vi "Main.vi"() -> ()   [LabVIEW 2022 SP3]
doc: "该连续测量范例项目在队列消息处理器模板的基础上实现。\n\n事件处理循环负责按用户界面操作生成对应的消息。\n\n消息处理循环负责对事件处理循环或其他消息生成的消息进行处理。 其中还包括用于采集和记录消息处理循环的子VI，以及用于更新图表的循环。"
uses:
  Settings/Settings.ctl
  Acquisition/Hardware Configuration.ctl
  Acquisition/Signal Type.ctl
  Logging/Logging Configuration.ctl
  controls/UI Data.ctl
  controls/UI State.ctl
  support/Message Queue/Enqueue Message (Single).vi
  support/Message Queue/Enqueue Message (Array).vi
  <vilib>/Utility/error.llb/Error Cluster From Error Code.vi
  <vilib>/ErrorRing/Error Ring.xnode
  Acquisition/Acquisition.lvlib
  Logging/Logging.lvlib
  Settings/Settings.lvlib
  support/User Event - Stop/User Event - Stop.lvlib
  support/Message Queue/Message Queue.lvlib
  Settings/Settings Dialog.vi
panel:
  out "数据":waveform(dbl)[](graph)
  in  "设置":bool
  in  "开始":bool
  in  "停止":bool
  out "状态":string
  in  "退出":bool
  # "连续测量数据记录器"
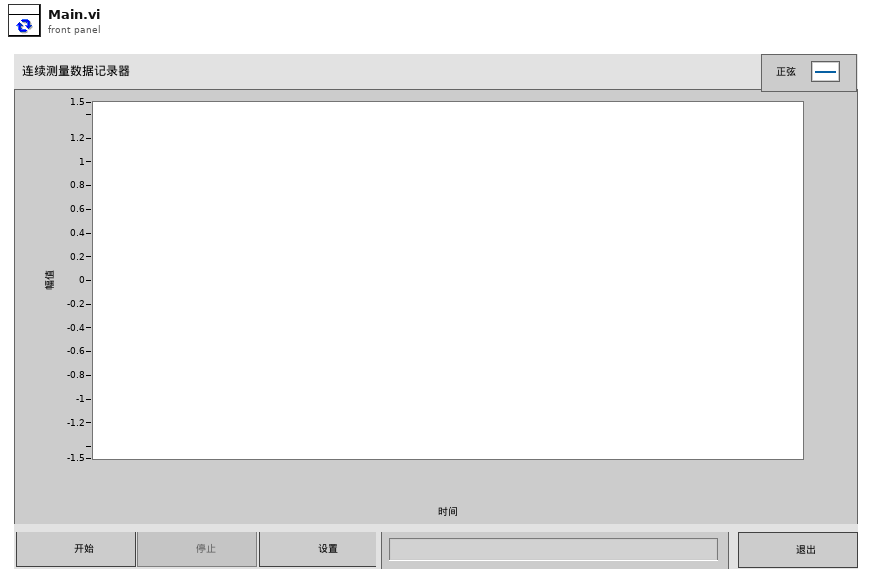
[diagram p1: front panel]
types:
  T1 = typedef "UI State.ctl" = enum16{"Idle", "Acquiring and Logging", "Waiting for Exit", "Waiting for Exit (Acq Stopped)", "Waiting for Exit (Log Stopped)", "Waiting for Stop", "Waiting for Stop (Acq Stopped)", "Waiting for Stop (Log Stopped)"}
  T2 = typedef "UI Data.ctl" = cluster{"开始引用":refnum<vi>, "停止引用":refnum<vi>, "设置引用":refnum<vi>, "退出引用":refnum<vi>, "状态引用":refnum<vi>, "数据引用":refnum<vi>}
  T3 = typedef "Settings.lvlib/Settings.ctl" = cluster{"硬件配置":T4, "记录配置":T6}
  T4 = typedef "Acquisition.lvlib/Hardware Configuration.ctl" = cluster{"硬件引用句柄<替换此项>":string, "信号类型<替换该项>":T5}
  T5 = typedef "Acquisition.lvlib/Signal Type.ctl" = enum16{"Sine Wave", "Square with Noise"}
  T6 = typedef "Logging.lvlib/Logging Configuration.ctl" = cluster{"记录文件基路径":path, "TDMS文件引用":refnum<k34>}
  T7 = typedef "Message Queue.lvlib/All Message Queues.ctl" = cluster{"UI":refnum<queue>, "采集":refnum<queue>, "记录":refnum<queue>}
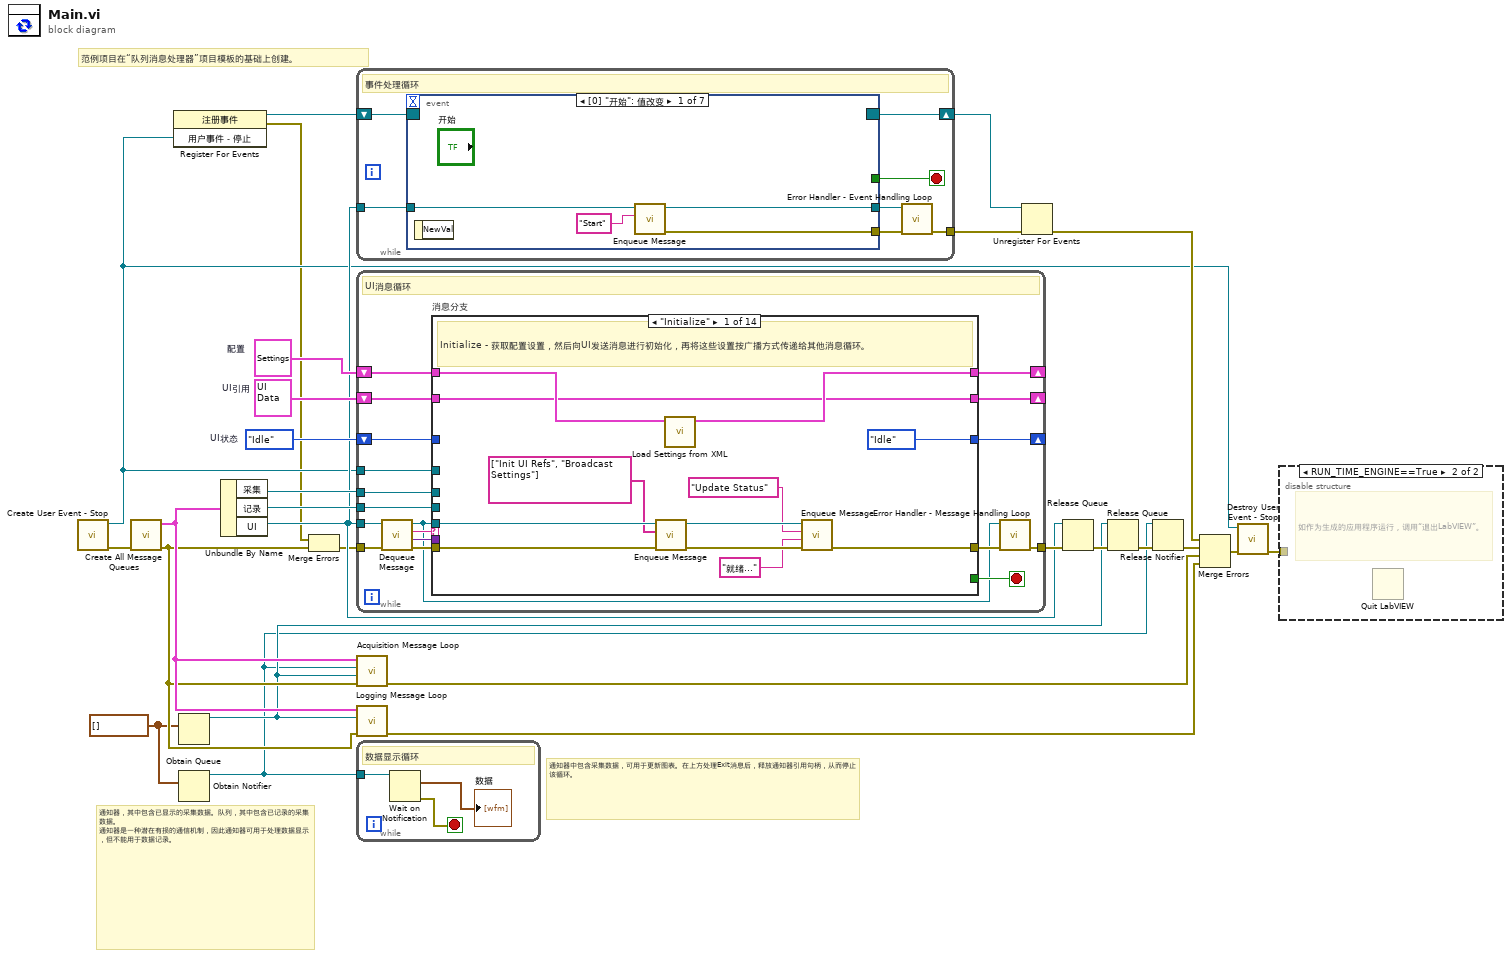
[diagram p0: block diagram]
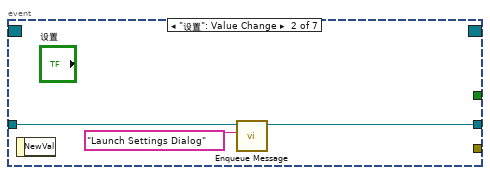
[diagram p3: hidden frame]
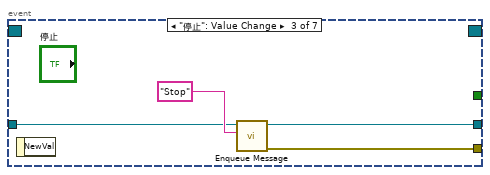
[diagram p4: hidden frame]
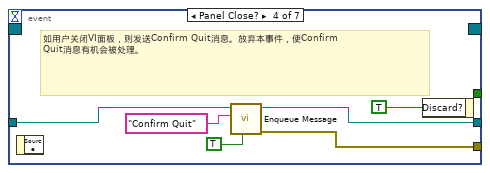
[diagram p5: hidden frame]
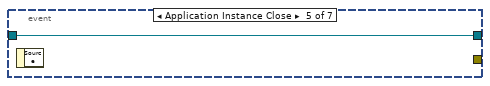
[diagram p6: hidden frame]
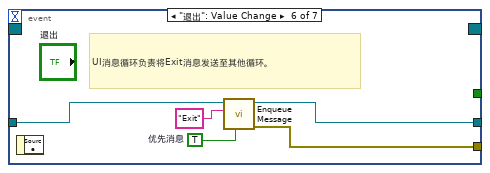
[diagram p7: hidden frame]
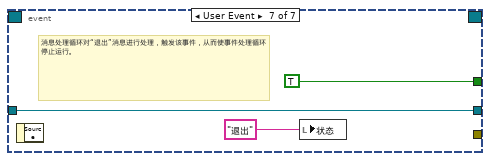
[diagram p8: hidden frame]
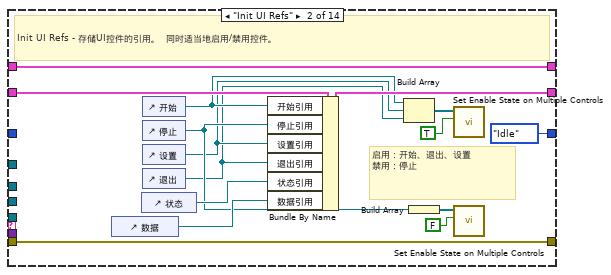
[diagram p9: hidden frame]
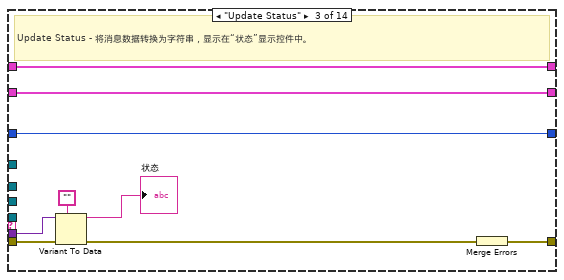
[diagram p10: hidden frame]
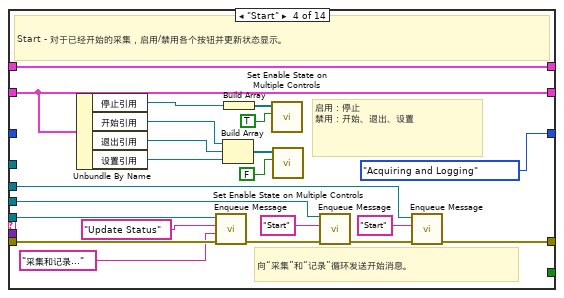
[diagram p11: hidden frame]
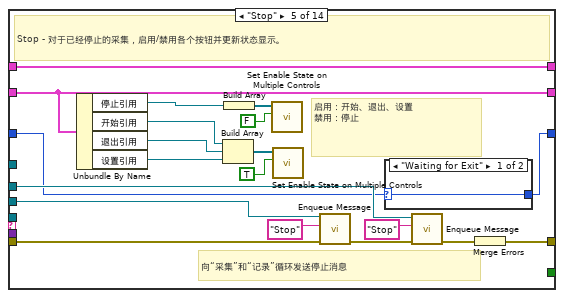
[diagram p12: hidden frame]
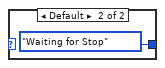
[diagram p13: hidden frame]
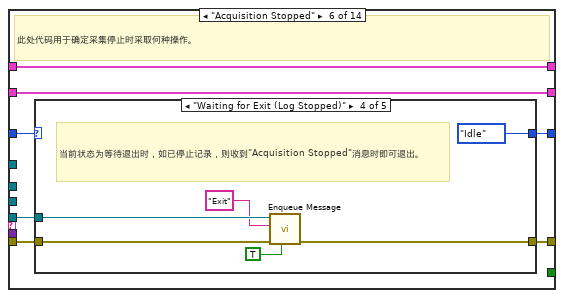
[diagram p14: hidden frame]
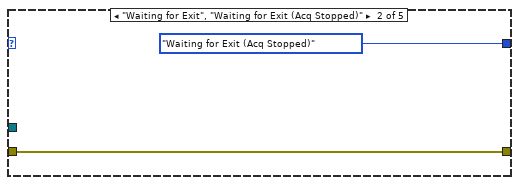
[diagram p16: hidden frame]
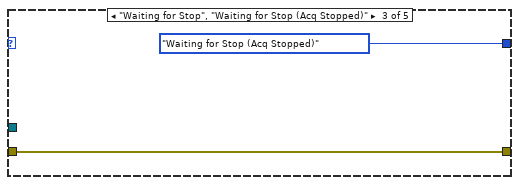
[diagram p17: hidden frame]
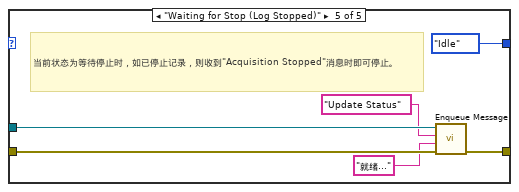
[diagram p18: hidden frame]
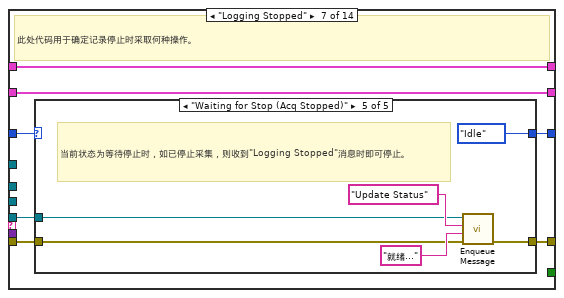
[diagram p19: hidden frame]
diagram:
  w14 = UI_State."Idle"  # UI状态
  w5 = waveform(dbl)[] []
  w17 = T2 {"开始引用"=refnum, "停止引用"=refnum, "设置引用"=refnum, "退出引用"=refnum, "状态引用"=refnum, "数据引用"=refnum}  # UI引用
  w20 = T3 {"硬件配置"={"硬件引用句柄<替换此项>"="", "信号类型<替换该项>"=enum."Sine Wave"}, "记录配置"={"记录文件基路径"=path "", "TDMS文件引用"=refnum}}  # 配置
  # "范例项目在“队列消息处理器”项目模板的基础上创建。"
  # "通知器，其中包含已显示的采集数据。队列，其中包含已记录的采集数据。  通知器是一种潜在有损的通信机制，因此通知器可用于处理数据显示，但不能用于数据记录。"
  # "通知器中包含采集数据，可用于更新图表。在上方处理Exit消息后，释放通知器引用句柄，从而停止该循环。"
  n1 = call "Create User Event - Stop.vi"() -> ("error out"=w24:cluster{"状态":bool, "代码":i32, "源":string}, "用户事件－停止"=w3:refnum<user-event>)  [unwired: 10 in]
  n2 = call "Create All Message Queues.vi"("error in (no error)"=w24) -> ("error out"=w21:cluster{"状态":bool, "代码":i32, "源":string}, "消息队列输出"=w23:T7)  [unwired: 9 in]
  n3 = register-events(w3) -> (reference out=w4:refnum<event-registration>, error out=w1:errorcluster)  [unwired: 2 in]
  n4 = Obtain Queue(element data type=w5) -> (queue out=w7:refnum<queue>)  [unwired: 4 in, 2 out]
  n5 = Obtain Notifier(notification data type=w5) -> (notifier out=w6:refnum<notifier>)  [unwired: 3 in, 2 out]
  n6 = Unbundle By Name(w23) -> ("采集"=w16:refnum<queue>, "记录"=w15:refnum<queue>, "UI"=w12:refnum<queue>)
  n7 = Merge Errors(w1, w21) -> (w2:errorcluster)
  n8 = while {
    tunnel: w12 -> [w33]
    tunnel: [w30] -> w26
    shift-right: [w32] -> w18
    shift-left: w4 -> [w34]
    stop <- w31 stop-if-true
    # "事件处理循环"
    n9 = event shown="[0] \"开始\": 值改变" {
      selector: w34 -> [_ _ _ _ _ _ _]
      dyn-events: [_ _ _ _ _ _ _] -> w32
      timeout: _ -> [_ _ _ _ _ _ _]
      tunnel: [_ _ _ _ _ _ TRUE ("Discard?")] -> w31
      tunnel: w33 -> [w38 w40 w44 w49 w52 w54 w58]
      tunnel: [w36 _ w43 w47 _ w57 _] -> w29
      tunnel: [w35 w39 w42 w48 w52 w53 w58] -> w28
      event "开始": Value Change {
        n10 = event-data() -> ()  [unwired: 1 in, 1 out]
        n11 = call-poly "Enqueue Message.vi"("消息"="Start" ("Message"), "消息队列"=w38) -> ("error out"=w36:cluster{"状态":bool, "代码":i32, "源":string}, "消息队列副本"=w35:refnum<queue>)  [unwired: 8 in]
      }
      event "设置": Value Change {
        n12 = event-data() -> ()  [unwired: 1 in, 1 out]
        n13 = call-poly "Enqueue Message.vi"("消息"="Launch Settings Dialog" ("Message"), "消息队列"=w40) -> ("消息队列副本"=w39:refnum<queue>)  [unwired: 8 in, 1 out]
      }
      event "停止": Value Change {
        n14 = event-data() -> ()  [unwired: 1 in, 1 out]
        n15 = call-poly "Enqueue Message.vi"("消息"="Stop" ("Message"), "消息队列"=w44) -> ("error out"=w43:cluster{"状态":bool, "代码":i32, "源":string}, "消息队列副本"=w42:refnum<queue>)  [unwired: 8 in]
      }
      event Panel Close? {
        # "如用户关闭VI面板，则发送Confirm Quit消息。放弃本事件，使Confirm Quit消息有机会被处理。"
        n16 = event-data() -> ()  [unwired: 1 in, 1 out]
        n17 = call-poly "Enqueue Message.vi"("优先消息？ (F)"=TRUE ("Priority Message? (F)"), "消息"="Confirm Quit" ("Message"), "消息队列"=w49) -> ("error out"=w47:cluster{"状态":bool, "代码":i32, "源":string}, "消息队列副本"=w48:refnum<queue>)  [unwired: 7 in]
        n18 = event-data ("Event Filter Node")("Discard?"=TRUE) -> ()  [unwired: 1 in, 1 out]
      }
      event Application Instance Close {
        n19 = event-data() -> ()  [unwired: 1 in, 1 out]
      }
      event "退出": Value Change {
        w55 = TRUE  # 优先消息
        # "UI消息循环负责将Exit消息发送至其他循环。"
        n20 = event-data() -> ()  [unwired: 1 in, 1 out]
        n21 = call-poly "Enqueue Message.vi"("优先消息？ (F)"=w55, "消息"="Exit" ("Message"), "消息队列"=w54) -> ("error out"=w57:cluster{"状态":bool, "代码":i32, "源":string}, "消息队列副本"=w53:refnum<queue>)  [unwired: 7 in]
      }
      event User Event {
        # "消息处理循环对“退出”消息进行处理，触发该事件，从而使事件处理循环停止运行。"
        n22 = event-data() -> ()  [unwired: 1 in, 1 out]
        n23 = local write "状态"("退出" ("Exit String")) -> ()
      }
    }
    n24 = call "Error Handler - Event Handling Loop.vi"("error in (no error)"=w29, "消息队列"=w28) -> ("错误输入副本"=w30:cluster{"状态":bool, "代码":i32, "源":string})  [unwired: 8 in, 1 out]
  }
  n25 = while {
    tunnel: w12 -> [w72]
    tunnel: w3 -> [w77]
    shift-right: [w71] -> _
    shift-left: w20 -> [w70]
    shift-right: [w68] -> _
    shift-left: w17 -> [w69]
    tunnel: w16 -> [w67]
    tunnel: w15 -> [w66]
    shift-right: [w61] -> _
    shift-left: w14 -> [w62]
    tunnel: w2 -> [w76]
    tunnel: [w65] -> w27
    stop <- w78 stop-if-true
    # "UI消息循环"
    n26 = call "Dequeue Message.vi"("error in (no error)"=w76, "消息队列"=w72) -> ("error out"=w75:cluster{"状态":bool, "代码":i32, "源":string}, "消息数据"=w73:variant, "消息"=w74:string, "消息队列副本"=w63:refnum<queue>)  [unwired: 6 in]
    n27 = case "消息分支" shown="\"Initialize\"" w74 {
      selector: w74 -> [_ _ _ _ _ _ _ _ _ _ _ _ _ w294]
      tunnel: w63 -> [w82 _ _ w136 _ w161 w186 _ w226 _ w247 _ _ _]
      tunnel: w75 -> [w81 w105 w113 w135 w155 w162 w187 w214 w228 w235 w246 w275 w292 _]
      tunnel: [w86 w105 w114 w118 w156 w159 w184 w220 w221 w238 w245 w285 w291 w293] -> w64
      tunnel: [_ _ _ _ _ _ _ _ _ _ _ TRUE _ _] -> w78
      tunnel: w73 -> [_ _ w112 _ _ _ _ _ _ w239 _ w273 _ _]
      tunnel: w77 -> [_ _ _ _ _ _ _ _ _ _ _ w286 _ _]
      tunnel: [w89 w104 w108 w134 w154 w165 w190 w218 w225 w243 w250 w284 w290 w297] -> w71
      tunnel: w70 -> [w90 w104 w108 w134 w154 w165 w190 w218 w229 w243 w250 w284 w290 w297]
      tunnel: w69 -> [w83 w103 w107 w131 w153 w164 w189 w212 w223 w242 w249 w283 w289 w296]
      tunnel: [w83 w100 w107 w131 w153 w164 w189 w212 w223 w242 w249 w283 w289 w296] -> w68
      tunnel: w67 -> [_ _ _ w117 w140 _ _ w211 _ _ _ w282 _ _]
      tunnel: w66 -> [_ _ _ w120 w143 _ _ w210 _ _ _ w281 _ _]
      tunnel: w62 -> [_ _ w106 _ w137 w163 w188 w209 w222 w237 w248 _ w288 w295]
      tunnel: [UI_State."Idle" ("UI State") UI_State."Idle" ("UI State") w106 UI_State."Acquiring and Logging" ("UI State") w138 w160 w185 w209 w222 w237 w244 UI_State."Idle" ("UI State") w288 w295] -> w61
      frame "Initialize" {
        # "Initialize - 获取配置设置，然后向UI发送消息进行初始化，再将这些设置按广播方式传递给其他消息循环。"
        n28 = call-poly "Enqueue Message.vi"("error in (no error)"=w81, "消息数组"=string[] ["Init UI Refs", "Broadcast Settings"], "消息队列"=w82) -> ("error out"=w88:cluster{"状态":bool, "代码":i32, "源":string}, "消息队列副本"=w87:refnum<queue>)  [unwired: 7 in]
        n29 = call "Load Settings from XML.vi"("设置输入"=w90) -> ("设置输出"=w89:T3)  [unwired: 9 in, 1 out]
        n30 = call-poly "Enqueue Message.vi"("error in (no error)"=w88, "消息数据"="就绪..." ("Ready..."), "消息"="Update Status" ("Message"), "消息队列"=w87) -> ("error out"=w86:cluster{"状态":bool, "代码":i32, "源":string})  [unwired: 6 in, 1 out]
      }
      frame "Init UI Refs" {
        # "启用：开始、退出、设置\n禁用：停止"
        # "Init UI Refs - 存储UI控件的引用。  同时适当地启用/禁用控件。"
        n31 = control-ref of="数据"() -> (w101:refnum<vi>)
        n32 = control-ref of="状态"() -> (w102:refnum<vi>)
        n33 = control-ref of="开始"() -> (w94:refnum<vi>)
        n34 = control-ref of="停止"() -> (w95:refnum<vi>)
        n35 = control-ref of="设置"() -> (w93:refnum<vi>)
        n36 = control-ref of="退出"() -> (w92:refnum<vi>)
        n37 = Bundle By Name(cluster=w103, "开始引用"=w94, "停止引用"=w95, "设置引用"=w93, "退出引用"=w92, "状态引用"=w102, "数据引用"=w101) -> (w100:T2)
        n38 = Build Array(w94, w93, w92) -> (w98:refnum<vi>[])
        n39 = Build Array(w95) -> (w97:refnum<vi>[])
        n40 = call "Set Enable State on Multiple Controls.vi"("启用？"=TRUE ("Enable?"), "控件"=w98) -> ()  [unwired: 10 in]
        n41 = call "Set Enable State on Multiple Controls.vi"("启用？"=FALSE ("Enable?"), "控件"=w97) -> ()  [unwired: 10 in]
      }
      frame "Update Status" {
        # "Update Status - 将消息数据转换为字符串，显示在“状态”显示控件中。"
        n42 = Variant To Data(error in=w113, type="" ("Empty String Constant"), Variant=w112) -> (data=→"状态":string, error out=w110:errorcluster)
        n43 = Merge Errors(w110) -> (w114:errorcluster)
      }
      frame "Start" {
        # "向“采集”和“记录”循环发送开始消息。"
        # "启用：停止\n禁用：开始、退出、设置"
        # "Start - 对于已经开始的采集，启用/禁用各个按钮并更新状态显示。"
        n44 = Unbundle By Name(w131) -> ("停止引用"=w126:refnum<vi>, "开始引用"=w125:refnum<vi>, "退出引用"=w124:refnum<vi>, "设置引用"=w123:refnum<vi>)
        n45 = call-poly "Enqueue Message.vi"("error in (no error)"=w135, "消息数据"="采集和记录..." ("Acquiring and Logging..."), "消息"="Update Status" ("Message"), "消息队列"=w136) -> ("error out"=w122:cluster{"状态":bool, "代码":i32, "源":string})  [unwired: 6 in, 1 out]
        n46 = Build Array(w125, w124, w123) -> (w129:refnum<vi>[])
        n47 = Build Array(w126) -> (w128:refnum<vi>[])
        n48 = call "Set Enable State on Multiple Controls.vi"("启用？"=TRUE ("Enable?"), "控件"=w128) -> ()  [unwired: 10 in]
        n49 = call "Set Enable State on Multiple Controls.vi"("启用？"=FALSE ("Enable?"), "控件"=w129) -> ()  [unwired: 10 in]
        n50 = call-poly "Enqueue Message.vi"("error in (no error)"=w122, "消息"="Start" ("Message"), "消息队列"=w120) -> ("error out"=w119:cluster{"状态":bool, "代码":i32, "源":string})  [unwired: 7 in, 1 out]
        n51 = call-poly "Enqueue Message.vi"("error in (no error)"=w119, "消息"="Start" ("Message"), "消息队列"=w117) -> ("error out"=w118:cluster{"状态":bool, "代码":i32, "源":string})  [unwired: 7 in, 1 out]
      }
      frame "Stop" {
        # "向“采集”和“记录”循环发送停止消息"
        # "启用：开始、退出、设置\n禁用：停止"
        # "Stop - 对于已经停止的采集，启用/禁用各个按钮并更新状态显示。"
        n52 = Unbundle By Name(w153) -> ("停止引用"=w148:refnum<vi>, "开始引用"=w147:refnum<vi>, "退出引用"=w146:refnum<vi>, "设置引用"=w145:refnum<vi>)
        n53 = Build Array(w147, w146, w145) -> (w151:refnum<vi>[])
        n54 = Build Array(w148) -> (w150:refnum<vi>[])
        n55 = call "Set Enable State on Multiple Controls.vi"("启用？"=FALSE ("Enable?"), "控件"=w150) -> ()  [unwired: 10 in]
        n56 = call "Set Enable State on Multiple Controls.vi"("启用？"=TRUE ("Enable?"), "控件"=w151) -> ()  [unwired: 10 in]
        n57 = call-poly "Enqueue Message.vi"("error in (no error)"=w155, "消息"="Stop" ("Message"), "消息队列"=w143) -> ("error out"=w142:cluster{"状态":bool, "代码":i32, "源":string})  [unwired: 7 in, 1 out]
        n58 = case shown="\"Waiting for Exit\"" w137 {
          selector: w137 -> [w157 _]
          tunnel: [w157 UI_State."Waiting for Stop" ("UI State")] -> w138
          frame "Waiting for Exit" {
          }
          frame Default {
          }
        }
        n59 = call-poly "Enqueue Message.vi"("error in (no error)"=w142, "消息"="Stop" ("Message"), "消息队列"=w140) -> ("error out"=w141:cluster{"状态":bool, "代码":i32, "源":string})  [unwired: 7 in, 1 out]
        n60 = Merge Errors(w141) -> (w156:errorcluster)
      }
      frame "Acquisition Stopped" {
        # "此处代码用于确定采集停止时采取何种操作。"
        n61 = case shown="\"Waiting for Exit (Log Stopped)\"" w163 {
          selector: w163 -> [w167 _ _ _ _]
          tunnel: w162 -> [w166 w169 w171 w177 w183]
          tunnel: w161 -> [_ _ _ w175 w180]
          tunnel: [w167 UI_State."Waiting for Exit (Acq Stopped)" ("UI State") UI_State."Waiting for Stop (Acq Stopped)" ("UI State") UI_State."Idle" ("UI State") UI_State."Idle" ("UI State")] -> w160
          tunnel: [w166 w169 w171 w176 w181] -> w159
          frame Default {
          }
          frame "Waiting for Exit", "Waiting for Exit (Acq Stopped)" {
          }
          frame "Waiting for Stop", "Waiting for Stop (Acq Stopped)" {
          }
          frame "Waiting for Exit (Log Stopped)" {
            # "当前状态为等待退出时，如已停止记录，则收到\"Acquisition Stopped\"消息时即可退出。"
            n62 = call-poly "Enqueue Message.vi"("优先消息？ (F)"=TRUE ("Priority Message? (F)"), "error in (no error)"=w177, "消息"="Exit", "消息队列"=w175) -> ("error out"=w176:cluster{"状态":bool, "代码":i32, "源":string})  [unwired: 6 in, 1 out]
          }
          frame "Waiting for Stop (Log Stopped)" {
            # "当前状态为等待停止时，如已停止记录，则收到\"Acquisition Stopped\"消息时即可停止。"
            n63 = call-poly "Enqueue Message.vi"("error in (no error)"=w183, "消息数据"="就绪..." ("Ready..."), "消息"="Update Status" ("Message"), "消息队列"=w180) -> ("error out"=w181:cluster{"状态":bool, "代码":i32, "源":string})  [unwired: 6 in, 1 out]
          }
        }
      }
      frame "Logging Stopped" {
        # "此处代码用于确定记录停止时采取何种操作。"
        n64 = case shown="\"Waiting for Stop (Acq Stopped)\"" w188 {
          selector: w188 -> [w192 _ _ _ _]
          tunnel: w187 -> [w191 w194 w196 w202 w205]
          tunnel: w186 -> [_ _ _ w200 w204]
          tunnel: [w192 UI_State."Waiting for Exit (Log Stopped)" ("UI State") UI_State."Waiting for Stop (Log Stopped)" ("UI State") UI_State."Idle" ("UI State") UI_State."Idle" ("UI State")] -> w185
          tunnel: [w191 w194 w196 w201 w203] -> w184
          frame Default {
          }
          frame "Waiting for Exit", "Waiting for Exit (Log Stopped)" {
          }
          frame "Waiting for Stop", "Waiting for Stop (Log Stopped)" {
          }
          frame "Waiting for Exit (Acq Stopped)" {
            # "当前状态为等待退出时，如已停止采集，则收到\"Logging Stopped\"消息时即可退出。"
            n65 = call-poly "Enqueue Message.vi"("优先消息？ (F)"=TRUE ("Priority Message? (F)"), "error in (no error)"=w202, "消息"="Exit", "消息队列"=w200) -> ("error out"=w201:cluster{"状态":bool, "代码":i32, "源":string})  [unwired: 6 in, 1 out]
          }
          frame "Waiting for Stop (Acq Stopped)" {
            # "当前状态为等待停止时，如已停止采集，则收到\"Logging Stopped\"消息时即可停止。"
            n66 = call-poly "Enqueue Message.vi"("error in (no error)"=w205, "消息数据"="就绪..." ("Ready..."), "消息"="Update Status" ("Message"), "消息队列"=w204) -> ("error out"=w203:cluster{"状态":bool, "代码":i32, "源":string})  [unwired: 6 in, 1 out]
          }
        }
      }
      frame "Broadcast settings" {
        w213 = "Update Settings" ("Message")
        # "Broadcast settings - 向“记录和采集”消息队列发送“更新设置”消息。"
        n67 = Unbundle By Name(w218) -> ("硬件配置"=w217:T4, "记录配置"=w216:T6)
        n68 = call-poly "Enqueue Message.vi"("消息数据"=w217, "消息"=w213, "消息队列"=w211) -> ("error out"=w219:cluster{"状态":bool, "代码":i32, "源":string})  [unwired: 7 in, 1 out]
        n69 = call-poly "Enqueue Message.vi"("error in (no error)"=w219, "消息数据"=w216, "消息"=w213, "消息队列"=w210) -> ("error out"=w215:cluster{"状态":bool, "代码":i32, "源":string})  [unwired: 6 in, 1 out]
        n70 = Merge Errors(w215, w214) -> (w220:errorcluster)
      }
      frame "Launch Settings Dialog" {
        # "Launch Settings Dialog - 用户单击“设置”按钮时，启动设置对话框。"
        n71 = call-by-ref "?"("error in (no error)"=w228, "Settings in"=w229) -> ("error out"=w224:errorcluster, "Cancelled?"=w227:bool, "Settings out"=w225:T3)  [unwired: 8 in, 3 out]
        n72 = case shown="假" w227 {
          tunnel: w226 -> [w233 _]
          tunnel: w224 -> [w232 w234]
          tunnel: [w231 w234] -> w221
          frame False {
            n73 = call-poly "Enqueue Message.vi"("error in (no error)"=w232, "消息"="Broadcast Settings" ("Message"), "消息队列"=w233) -> ("error out"=w231:cluster{"状态":bool, "代码":i32, "源":string})  [unwired: 7 in, 1 out]
          }
          frame True {
          }
        }
      }
      frame "Error" {
        # "错误 - 显示错误对话框。该消息由本应用程序中其他循环结束处的“错误处理”VI发送。"
        n74 = Variant To Data(error in=w235, type=errorcluster {"status"=FALSE, "code"=0, "source"=""} ("error constant"), Variant=w239) -> (data=w236:errorcluster, error out=w240:errorcluster)
        n75 = call <vilib>:"Simple Error Handler.vi"("error in (no error)"=w236) -> ()  [unwired: 4 in, 5 out]
        n76 = Merge Errors(w240) -> (w238:errorcluster)
      }
      frame "Confirm Quit" {
        # "Confirm Quit - 该消息用于确认用户是否需要退出应用程序。"
        n77 = case shown="\"Acquiring and Logging\"" w248 {
          tunnel: w247 -> [w256 w260]
          tunnel: w246 -> [w255 w259]
          tunnel: [w254 w258] -> w245
          tunnel: [UI_State."Idle" ("UI State") w257] -> w244
          frame Default {
            # "如收到'Confirm Quit'消息时系统处于空闲状态，则不需要弹出确认提示。"
            n78 = call-poly "Enqueue Message.vi"("优先消息？ (F)"=TRUE ("Priority Message? (F)"), "error in (no error)"=w255, "消息"="Exit", "消息队列"=w256) -> ("error out"=w254:cluster{"状态":bool, "代码":i32, "源":string})  [unwired: 6 in, 1 out]
          }
          frame "Acquiring and Logging" {
            n79 = Two Button Dialog(message="采集仍在执行中，是否确定退出？" ("Confirm Quit Message"), 1:"否" ("No"), 2:"是" ("Yes")) -> (T button?=w261:bool)
            n80 = case shown="真" w261 {
              tunnel: w260 -> [_ w270]
              tunnel: w259 -> [w266 w271]
              tunnel: [w266 w269] -> w258
              tunnel: [UI_State."Acquiring and Logging" ("UI State") UI_State."Waiting for Exit" ("UI State")] -> w257
              frame False {
                # "用户不希望退出。"
              }
              frame True {
                n81 = call-poly "Enqueue Message.vi"("error in (no error)"=w271, "消息"="Stop", "消息队列"=w270) -> ("error out"=w269:cluster{"状态":bool, "代码":i32, "源":string})  [unwired: 7 in, 1 out]
              }
            }
          }
        }
      }
      frame "Exit" {
        w277 = TRUE ("Priority Message? (F)")
        w278 = "Exit" ("Message")
        # "如果“Exit”为由于错误被调用，则弹出错误对话框。"
        # "停止VI"
        # "Exit - 发送“退出”消息至采集和记录循环，并触发用户事件停止事件处理循环。"
        n82 = Variant To Data(type=errorcluster {"status"=FALSE, "code"=0, "source"=""} ("error constant"), Variant=w273) -> (data=w272:errorcluster)  [unwired: 1 in, 1 out]
        n83 = call <vilib>:"Simple Error Handler.vi"("error in (no error)"=w272) -> ()  [unwired: 4 in, 5 out]
        n84 = call-poly "Enqueue Message.vi"("优先消息？ (F)"=w277, "error in (no error)"=w275, "消息"=w278, "消息队列"=w282) -> ("error out"=w279:cluster{"状态":bool, "代码":i32, "源":string})  [unwired: 6 in, 1 out]
        n85 = call-poly "Enqueue Message.vi"("优先消息？ (F)"=w277, "error in (no error)"=w279, "消息"=w278, "消息队列"=w281) -> ("error out"=w276:cluster{"状态":bool, "代码":i32, "源":string})  [unwired: 6 in, 1 out]
        n86 = call "Fire User Event - Stop.vi"("error in (no error)"=w276, "用户事件－停止"=w286) -> ("error out"=w285:cluster{"状态":bool, "代码":i32, "源":string})  [unwired: 9 in]
      }
      frame "---Copy This Frame---" {
        # "如需创建新消息，可创建该帧的副本。  在副本中，将本注释更改为对应消息的注释。"
        n87 = Merge Errors(w292) -> (w291:errorcluster)
      }
      frame Default {
        # "如得到的消息未经任何分支定义，则运行“默认”分支。  输出程序错误。"
        n88 = xnode ("Error Ring")("参数 0"=w294) -> ("错误输出"=w293:errorcluster)
      }
    }
    n89 = call "Error Handler - Message Handling Loop.vi"("error in (no error)"=w64, "消息队列"=w63) -> ("错误输入副本"=w65:cluster{"状态":bool, "代码":i32, "源":string})  [unwired: 8 in, 1 out]
  }
  n90 = call "Acquisition Message Loop.vi"("error in (no error)"=w21, "数据队列"=w7, "数据通知器"=w6, "消息队列"=w23) -> ("error out"=w25:cluster{"状态":bool, "代码":i32, "源":string})  [unwired: 7 in]
  n91 = call "Logging Message Loop.vi"("error in (no error)"=w21, "数据队列"=w7, "消息队列"=w23) -> ("error out"=w22:cluster{"状态":bool, "代码":i32, "源":string})  [unwired: 8 in]
  n92 = while "Data Display Loop" {
    tunnel: w6 -> [w307]
    stop <- w305 stop-if-true
    # "数据显示循环"
    n93 = Wait on Notification(notifier=w307) -> (notification=→"数据":waveform(dbl)[], error out=w305:errorcluster)  [unwired: 3 in, 2 out]
  }
  n94 = Unregister For Events(event registration refnum=w18, error in=w26) -> (error out=w19:errorcluster)
  n95 = Release Queue(queue=w12, error in (no error)=w27) -> (error out=w10:errorcluster)  [unwired: 1 in, 2 out]
  n96 = Release Queue(queue=w7, error in (no error)=w10) -> (error out=w9:errorcluster)  [unwired: 1 in, 2 out]
  n97 = Release Notifier(notifier=w6, error in (no error)=w9) -> (error out=w8:errorcluster)  [unwired: 1 in, 2 out]
  n98 = Merge Errors(w19, w8, w25, w22) -> (w13:errorcluster)
  n99 = call "Destroy User Event - Stop.vi"("error in (no error)"=w13, "用户事件－停止"=w3) -> ("error out"=w11:cluster{"状态":bool, "代码":i32, "源":string})  [unwired: 9 in]
  n100 = disable-structure "Conditional Disable Structure" shown="RUN_TIME_ENGINE==True" {
    disable-tunnel: w11 -> [_ _]
    frame condition #0 (active) {
    }
    frame condition #1 {
      # "如作为生成的应用程序运行，调用“退出LabVIEW”。"
      n101 = Quit LabVIEW() -> ()  [unwired: 1 in]
    }
  }
